vi "Reset.vi"(8 "error in (no error)":errorcluster, 11 "JMETestSolutions.Instrument in":refnum<class "JMETestSolutions.Instrument.lvclass">) -> (0 "error out":errorcluster, 3 "JMETestSolutions.Instrument out":refnum<class "JMETestSolutions.Instrument.lvclass">)   [LabVIEW 2020, in "JMETestSolutions.Instrument.lvlib" / "JMETestSolutions.Instrument.lvclass"]
doc: "Reset the Instrument to a known good state"
uses:
  JMETestSolutions.Instrument.lvclass
  JMETestSolutions.Instrument.lvclass/JMETestSolutions.Instrument.ctl
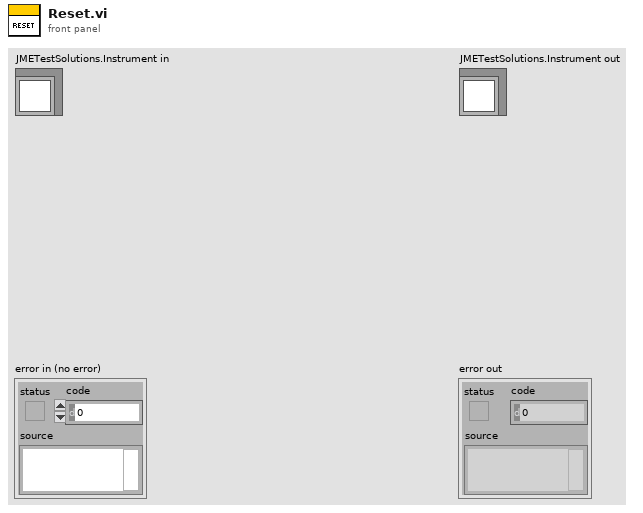
[diagram p1: front panel]
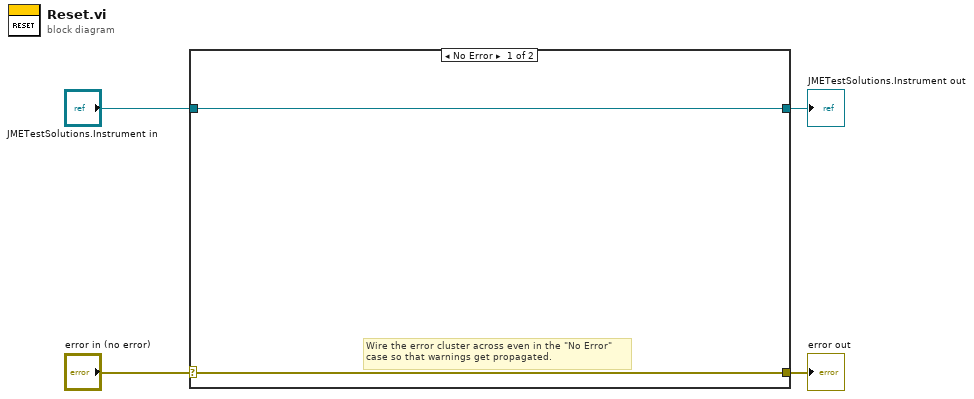
[diagram p0: block diagram]
diagram:
  n1 = case shown="No Error" "error in (no error)" {
    selector: "error in (no error)" -> [w5 w8]
    tunnel: [w5 w8] -> w3
    tunnel: [w6 w7] -> w1
    tunnel: "JMETestSolutions.Instrument in" -> [w6 w7]
    frame No Error {
      # "Wire the error cluster across even in the \"No Error\"\ncase so that warnings get propagated."
    }
    frame Error {
    }
  }
  "error out" <- w3
  "JMETestSolutions.Instrument out" <- w1
